vi "Do.vi"(10 "Y":dbl, 11 "X":dbl) -> (3 "Result":dbl)   [LabVIEW 2020, in "Add.lvlib"]
uses:
  Add.lvlib
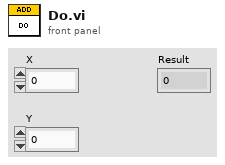
[diagram p1: front panel]
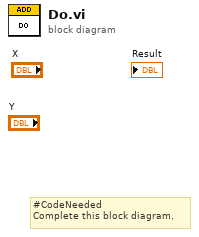
[diagram p0: block diagram]
diagram:
  # "#CodeNeeded\nComplete this block diagram."
